vi "CreatePublicEvents.vi"(8 "error in (no error)":errorcluster, 11 "SMO.UI":refnum<class "SMO.UI.lvclass">) -> (0 "error out":errorcluster, 3 "SMO.UI out":refnum<class "SMO.UI.lvclass">)   [LabVIEW 2019, in "SMO.UI.lvclass"]
doc: "JKI State Machine Objects (SMO) 1.3.0.56\nJKI - JKI\nCopyright (c) 2017, JKI"
uses:
  SMO.UI.lvclass
  SMO.UI.lvclass/SMO.UI.ctl
  Typedefs/SMO.UI State--enum.ctl
  SMO/SMO.lvclass
panel:
  # "For instructions on how to use the JKI State Machine Objects, examples and video tutorials, visit:\nhttp://jki.net/state-machine-objects/\n\nJKI State Machine Objects™\nhttp://jki.net/state-machine-objects/\nCopyright (C) 2005-2015, JKI <info@jki.net>\nALL RIGHTS RESERVED"
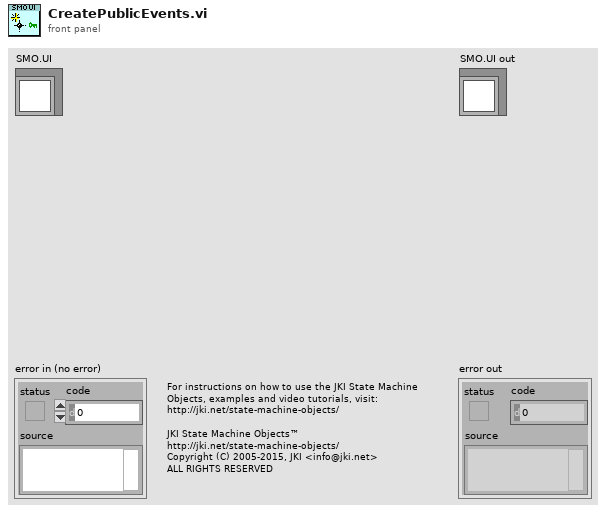
[diagram p1: front panel]
types:
  T1 = typedef "SMO.UI.lvclass/SMO.UI State--enum.ctl" = enum16{"unknown", "Opened", "Closed"}
  T2 = typedef "SMO.UI.lvclass/PrivateData--Ref.ctl" = refnum<data-value>
  T3 = cluster{"UI Closed":refnum<user-event>, "UI State":refnum<user-event>}
  T4 = typedef "SMO.UI.lvclass/PrivateData--Cluster.ctl" = cluster{"Public Events":T5, "Private Events":T6}
  T5 = typedef "SMO.UI.lvclass/PublicEvents--Cluster.ctl" = cluster{"UI Hidden":refnum<user-event>, "UI State":refnum<user-event>}
  T6 = typedef "SMO.UI.lvclass/PrivateEvents--Cluster.ctl" = cluster{"Show-Hide UI":refnum<user-event>}
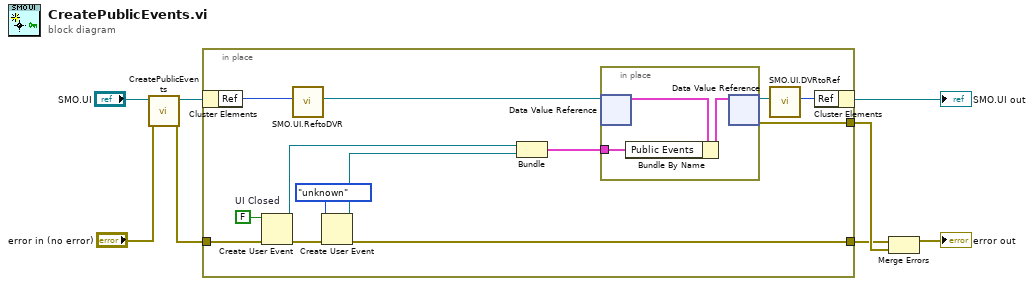
[diagram p0: block diagram]
diagram:
  n1 = call-parent "CreatePublicEvents.vi"("error in (no error)"="error in (no error)", "SMO"="SMO.UI") -> ("error out"=w2:errorcluster, "SMO out"=w3:refnum<class "SMO.UI.lvclass">)  [unwired: 8 in]
  n2 = in-place {
    in-place-border: [w21] -> w8
    in-place-border: w2 -> [w17]
    in-place-border: [w11] -> w1
    w18 = FALSE  # UI Closed
    n3 = in-place-cluster #1(w3) -> ("Ref"=w20:u32)
    n4 = Create User Event(user event datatype=w18, error in=w17) -> (user event=w13:refnum<user-event>, error out=w12:errorcluster)
    n5 = call "SMO.UI.ReftoDVR.vi"("Ref"=w20) -> ("Ref"=w19:T2)  [unwired: 10 in]
    n6 = Create User Event(user event datatype=SMO.UI_State--enum."unknown" ("UI State"), error in=w12) -> (user event=w10:refnum<user-event>, error out=w11:errorcluster)
    n7 = Bundle("UI Closed"=w13, "UI State"=w10) -> (w16:T3)  [unwired: 1 in]
    n8 = in-place {
      in-place-border: w16 -> [w22]
      n9 = in-place-dvr #2(w19) -> (w24:T4)  [unwired: 1 out]
      n10 = Bundle By Name(cluster=w24, "Public Events"=w22) -> (w23:T4)
      n11 = in-place-dvr #2(w23) -> (w15:T2, w21:errorcluster)
    }
    n12 = call "SMO.UI.DVRtoRef.vi"("Ref"=w15) -> ("Ref"=w14:u32)  [unwired: 10 in]
    n13 = in-place-cluster #1("Ref"=w14) -> (→"SMO.UI out":refnum<class "SMO.UI.lvclass">)
  }
  n14 = Merge Errors(w1, w8) -> (→"error out":errorcluster)
